vi "dfd_nMAC_AddNwLoad.vi"(0 "initIdx":fxp<+,16,16>, 3 "load":bool, 4 "step":fxp<+,16,16>) -> (7 "idxOut":fxp<+,16,16>)   [LabVIEW 2017]
uses:
  <vilib>/rvi/FXPMathLib/basic elements/FxpAddSub/XNode/nifxpmath_AddSub.xnode
  <vilib>/rvi/FXPMathLib/sim/FxpSim.dll
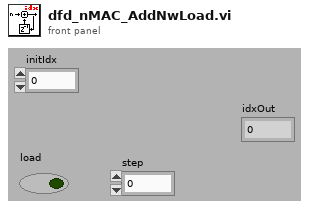
[diagram p1: front panel]
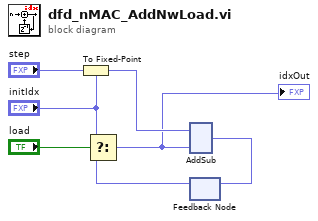
[diagram p0: block diagram]
diagram:
  n1 = To Fixed-Point(fixed-point type="initIdx", number="step") -> (fixed-point=w3:fxp<+,16,16>)
  n2 = feedback #1() -> (w4:fxp<+,16,16>)  [unwired: 1 out]
  n3 = Select(t="initIdx", s="load", f=w4) -> (s? t:f=w2:fxp<+,16,16>)
  "idxOut" <- w2
  n4 = xnode "AddSub"("x"=w3, "y"=w2) -> ("s"=w5:fxp<+,16,16>)  [unwired: 1 out]
  n5 = feedback-in #1(w5) -> ()
